vi "SendAO.vi"(5 "Message Priority (Normal)":T1=enum."Normal", 6 "StreamValue":T2, 7 "StaticValue":dbl, 8 "error in (no error)":errorcluster, 9 "OutChannel":u8, 10 "AoType":T3, 11 "Message Enqueuer":refnum<class "Message Enqueuer.lvclass">) -> (0 "error out":errorcluster)   [LabVIEW 2024, in "AIO Actor.lvlib" / "AIO Actor Msg.lvclass"]
uses:
  AIO Actor Msg.lvclass
  AO Type.ctl
  <vilib>/ActorFramework/Message Enqueuer/Message Enqueuer.lvclass
  <vilib>/ActorFramework/Message Enqueuer/Message Priority.ctl
  C:/Program Files (x86)/National Instruments/LabVIEW 2024/vi.lib/ActorFramework/Message/Message.lvclass
  AIO Actor Msg.lvclass/AIO Actor Msg.ctl
  <vilib>/ActorFramework/Message Enqueuer/Message Enqueuer.lvclass/Message Enqueuer.ctl
  <vilib>/ActorFramework/Message Priority Queue/Priority Enqueue.vi
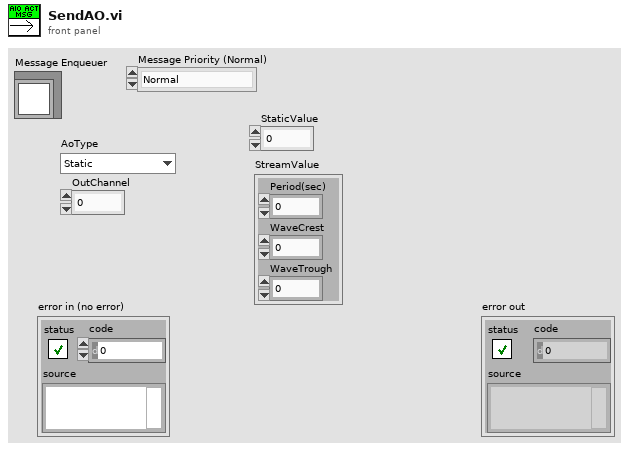
[diagram p1: front panel]
types:
  T1 = typedef "Actor Framework.lvlib/Message Enqueuer.lvclass/Message Priority.ctl" = enum16{"Low", "Normal", "High"}
  T2 = cluster{"Period(sec)":dbl, "WaveCrest":dbl, "WaveTrough":dbl}
  T3 = typedef "AO Type.ctl" = enum16{"Static", "Streaming", "StopStreaming"}
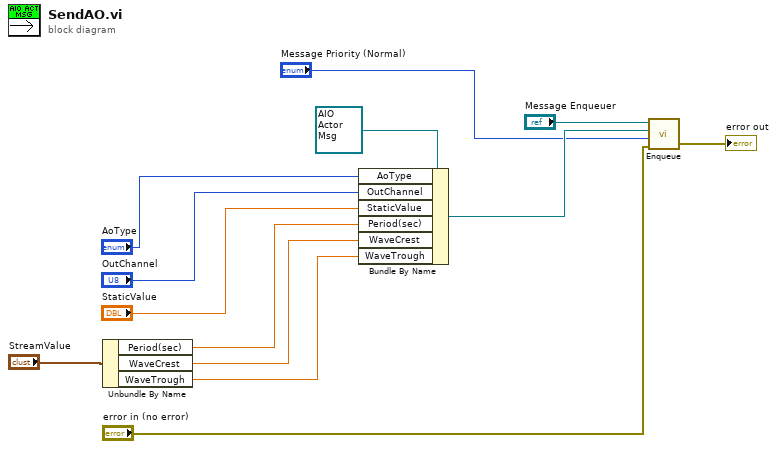
[diagram p0: block diagram]
diagram:
  n1 = Unbundle By Name("StreamValue") -> ("Period(sec)"=w7:dbl, "WaveCrest"=w6:dbl, "WaveTrough"=w5:dbl)
  n2 = Bundle By Name(cluster=refnum<class "AIO Actor Msg.lvclass"> refnum ("AIO Actor.lvlib:AIO Actor Msg.lvclass"), "AoType"="AoType", "OutChannel"="OutChannel", "StaticValue"="StaticValue", "Period(sec)"=w7, "WaveCrest"=w6, "WaveTrough"=w5) -> (w4:refnum<class "AIO Actor Msg.lvclass">)
  n3 = call <vilib>:"Enqueue.vi"("error in (no error)"="error in (no error)", "Message Priority (Normal)"="Message Priority (Normal)", "Message"=w4, "Message Enqueuer in"="Message Enqueuer") -> ("error out"=→"error out":errorcluster)  [unwired: 6 in, 1 out]
